vi "exercicio 4.vi"() -> ()   [LabVIEW 2025]
panel:
  out "Waveform Chart":dbl(graph)
  in  "Numeric 3":i32
  in  "stop 2":bool
  out "Numeric 2":i32
  in  "milliseconds to wait 2":u32
  out "x*y 2":dbl
  in  "F 2":dbl(slide) scale=0.0..212.0
  out "C 2":dbl(slide) scale=-100.0..100.0
  in  "Boolean":bool
  in  "F":dbl(slide) scale=0.0..212.0
  out "C":dbl(slide) scale=-100.0..100.0
  out "x*y":dbl
  in  "milliseconds to wait":u32
  out "Numeric":i32
  in  "stop":bool
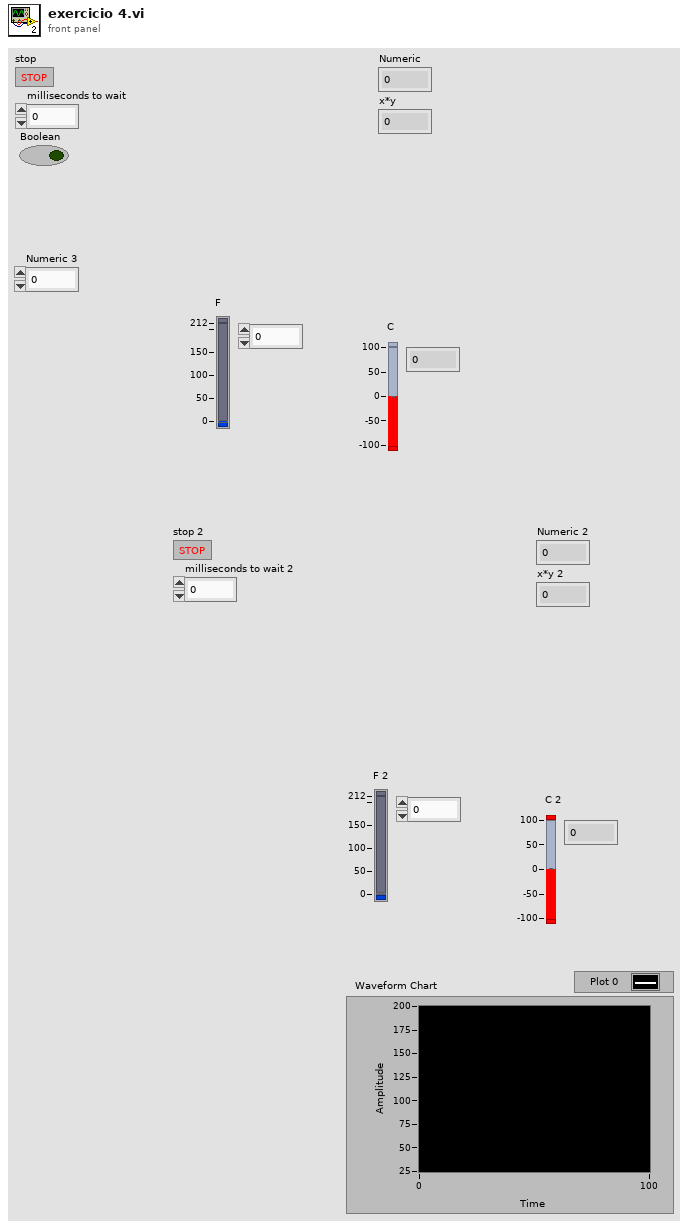
[diagram p1: front panel]
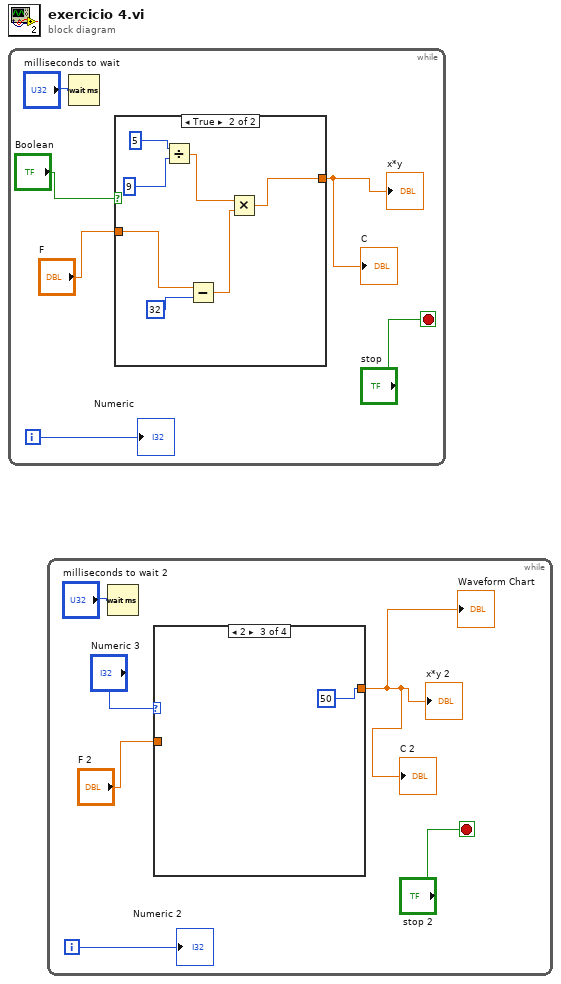
[diagram p0: block diagram]
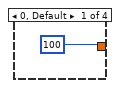
[diagram p2: hidden frame]
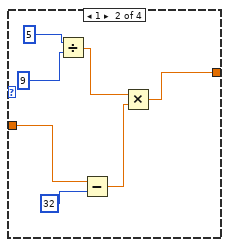
[diagram p3: hidden frame]
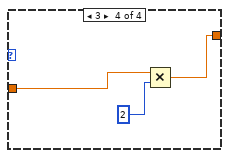
[diagram p4: hidden frame]
diagram:
  n1 = while {
    i -> [w4]
    stop <- "stop" stop-if-true
    n2 = Wait (ms)(milliseconds to wait="milliseconds to wait") -> ()  [unwired: 1 out]
    n3 = case shown="True" "Boolean" {
      tunnel: [w7 w9] -> w1
      tunnel: "F" -> [w7 w8]
      frame False {
      }
      frame True {
        n4 = Divide(x=5, y=9) -> (x/y=w12:dbl)
        n5 = Subtract(x=w8, y=32) -> (x-y=w10:dbl)
        n6 = Multiply(x=w12, y=w10) -> (x*y=w9:dbl)
      }
    }
    "x*y" <- w1
    "C" <- w1
    "Numeric" <- w4
  }
  n7 = while {
    i -> [w18]
    stop <- "stop 2" stop-if-true
    n8 = Wait (ms)(milliseconds to wait="milliseconds to wait 2") -> ()  [unwired: 1 out]
    n9 = case shown="2" "Numeric 3" {
      tunnel: [100 w23 50 w30] -> w15
      tunnel: "F 2" -> [_ w22 _ w32]
      frame 0, Default {
      }
      frame 1 {
        n10 = Divide(x=5, y=9) -> (x/y=w26:dbl)
        n11 = Subtract(x=w22, y=32) -> (x-y=w24:dbl)
        n12 = Multiply(x=w26, y=w24) -> (x*y=w23:dbl)
      }
      frame 2 {
      }
      frame 3 {
        n13 = Multiply(x=w32, y=2) -> (x*y=w30:dbl)
      }
    }
    "x*y 2" <- w15
    "C 2" <- w15
    "Waveform Chart" <- w15
    "Numeric 2" <- w18
  }
